vi "System Options.vi"(7 "Results Displayed (2:Last)":u16(ring)=2 items=["All", "Pass / Fail", "Last"], 8 "error in (no error)":errorcluster, 9 "Alarm Volume (5)":i32=5 min=0 max=9, 10 "Contrast (5)":i32=5 min=0 max=9, 11 "VISA resource name":refnum<visa-resource-name>) -> (0 "error out":errorcluster, 3 "VISA resource name out":refnum<visa-resource-name>)   [LabVIEW 2014, in "eec 6700.lvlib"]
doc: "Configures system options like Results format, LCD Display contrast, Step prompt, Alarm volume."
uses:
  <instrlib>/eec 6700/eec 6700.lvlib
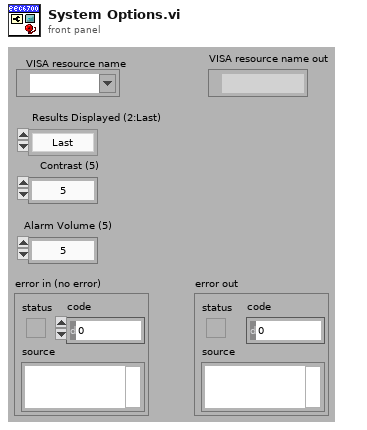
[diagram p1: front panel]
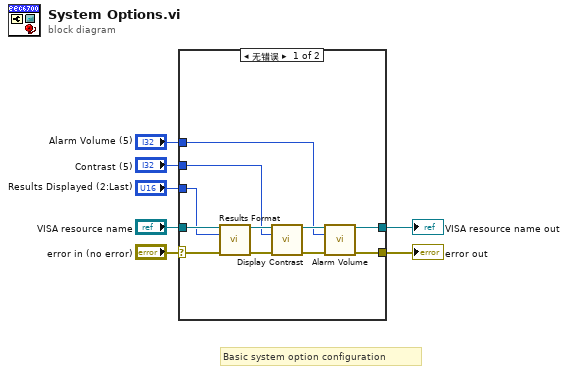
[diagram p0: block diagram]
diagram:
  # "Basic system option configuration"
  n1 = case shown="无错误" "error in (no error)" {
    selector: "error in (no error)" -> [w18 w20]
    tunnel: [w8 w20] -> w6
    tunnel: [w9 w19] -> w5
    tunnel: "VISA resource name" -> [w15 w19]
    tunnel: "Alarm Volume (5)" -> [w12 _]
    tunnel: "Contrast (5)" -> [w11 _]
    tunnel: "Results Displayed (2:Last)" -> [w10 _]
    frame No Error {
      n2 = call <instrlib>:"Results Format.vi"("VISA resource name"=w15, "Results Displayed (2:Last)"=w10, "error in (no error)"=w18) -> ("VISA resource name out"=w13:refnum<visa-resource-name>, "error out"=w17:errorcluster)  [unwired: 11 in]
      n3 = call <instrlib>:"Display Contrast.vi"("VISA resource name"=w13, "Contrast (5)"=w11, "error in (no error)"=w17) -> ("VISA resource name out"=w14:refnum<visa-resource-name>, "error out"=w16:errorcluster)  [unwired: 11 in]
      n4 = call <instrlib>:"Alarm Volume.vi"("VISA resource name"=w14, "Alarm Volume (5)"=w12, "error in (no error)"=w16) -> ("VISA resource name out"=w9:refnum<visa-resource-name>, "error out"=w8:errorcluster)  [unwired: 11 in]
    }
    frame Error {
    }
  }
  "VISA resource name out" <- w5
  "error out" <- w6
